vi "PICO init.vi"(8 "error in (no error)":errorcluster, 10 "Mains Frequency":i16(ring) items=["50 Hz", "60 Hz"], 11 "Digital in":refnum<vi>) -> (0 "error in (no error) 2":errorcluster, 3 "Handle":i16)   [LabVIEW 2015]
uses:
  Program Files (x86)/Pico Technology/SDK/lib/usbtc08.dll
panel:
  in  "Type # 1":i16(ring)=107 items=["B"=98, "E"=101, "J"=106, "K"=107, "N"=110, "R"=114, "S"=115, "T"=116, "Voltage"=120]
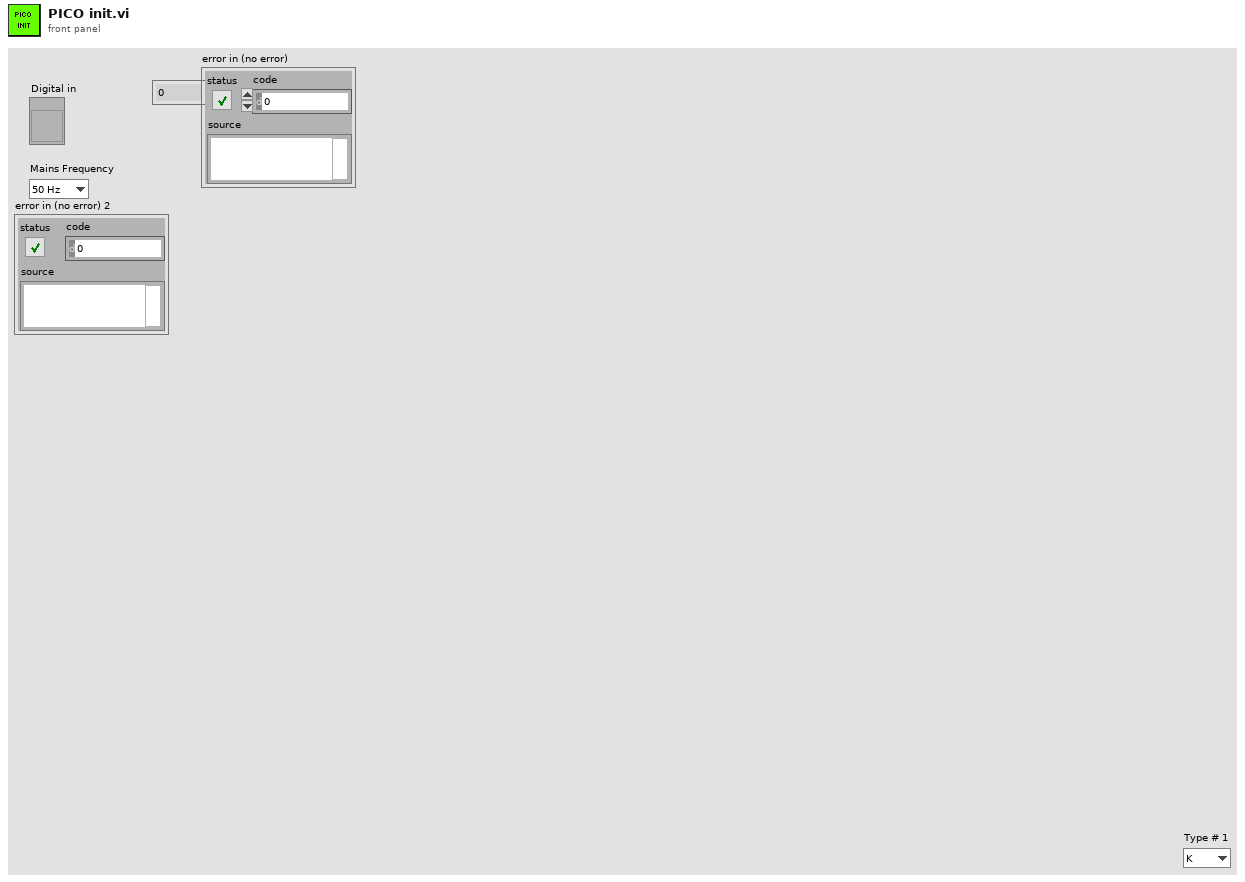
[diagram p1: front panel]
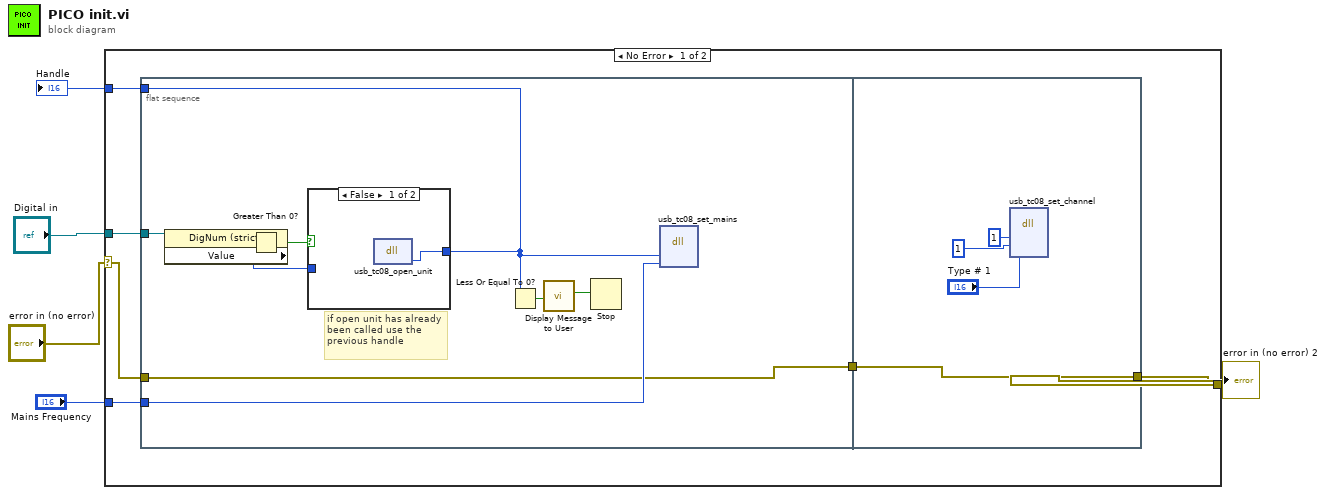
[diagram p0: block diagram]
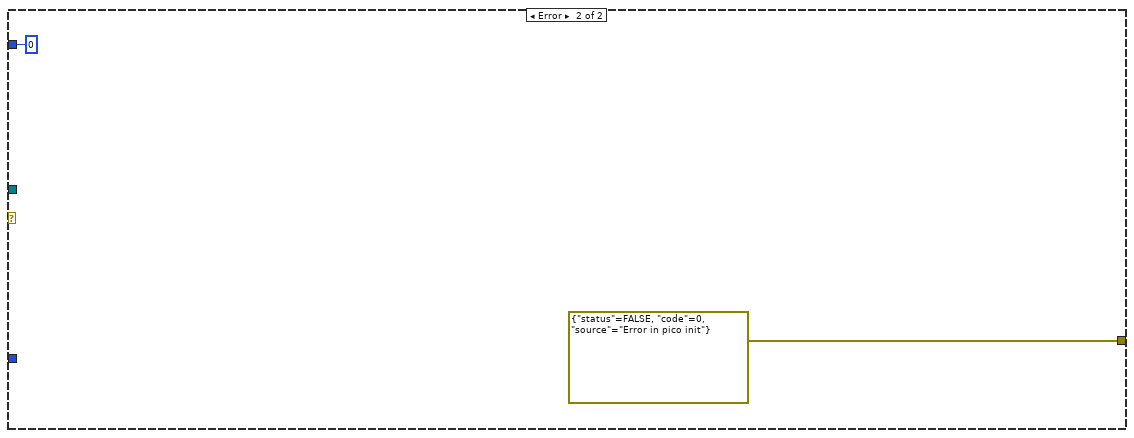
[diagram p3: hidden frame]
diagram:
  n1 = case shown="No Error" "error in (no error)" {
    selector: "error in (no error)" -> [w6 _]
    tunnel: "Mains Frequency" -> [w11 _]
    tunnel: [w10 i16 0 ("Value")] -> w4
    tunnel: "Digital in" -> [w9 _]
    tunnel: [w8 errorcluster {"status"=FALSE, "code"=0, "source"="Error in pico init"} ("error IO")] -> w1
    frame No Error {
      n2 = flat-sequence {
        tunnel: w11 -> [w19]
        tunnel: [w16] -> w10
        tunnel: w9 -> [w13]
        tunnel: [w12] -> w7
        tunnel: w6 -> [w12]
        tunnel: [w22] -> w8
        tunnel: w7 -> [w22]
        frame #0 {
          # "if open unit has already been called use the previous handle"
          n3 = property class="DigNum (strict)"(reference=w13) -> ("Value"=w15:i16)  [unwired: 1 in, 2 out]
          n4 = Greater Than 0?(x=w15) -> (x > 0?=w14:bool)
          n5 = case shown="False" w14 {
            tunnel: [w20 w21] -> w16
            tunnel: w15 -> [_ w21]
            frame False {
              n6 = dll-call lib="C:/Program Files (x86)/Pico Technology/SDK/lib/usbtc08.dll" fn="usb_tc08_open_unit" label="OpenUnit"() -> ("Handle"=w20:i16)  [unwired: 3 in, 2 out]
            }
            frame True {
            }
          }
          n7 = Less Or Equal To 0?(x=w16) -> (x <= 0?=w17:bool)
          n8 = call "Display Message to User"("Enable"=w17) -> ("OK"=w18:bool)  [unwired: 9 in, 1 out]
          n9 = Stop(stop? (T)=w18) -> ()
          n10 = dll-call lib="C:/Program Files (x86)/Pico Technology/SDK/lib/usbtc08.dll" fn="usb_tc08_set_mains" label="Set Mains"("Handle"=w16, "sixtyHertz"=w19) -> ()  [unwired: 6 in, 2 out]
        }
        frame #1 {
          n11 = dll-call lib="usbtc08.dll" fn="usb_tc08_set_channel"("handle"=i16 1, "channel"=i16 1, "tc_type"="Type # 1") -> ()  [unwired: 7 in, 2 out]
        }
      }
    }
    frame Error {
    }
  }
  "Handle" <- w4
  "error in (no error) 2" <- w1
